vi "UIntToDouble.vi"(1 "Value":u32, 2 "Max":dbl, 3 "Min":dbl) -> (0 "Number":dbl)   [LabVIEW 2009]
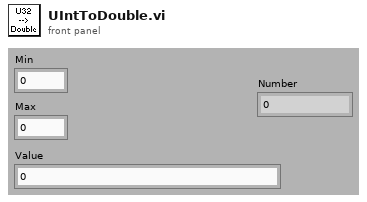
[diagram p1: front panel]
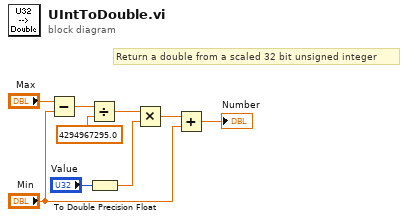
[diagram p0: block diagram]
diagram:
  # "Return a double from a scaled 32 bit unsigned integer"
  n1 = Subtract(x="Max", y="Min") -> (x-y=w9:dbl)
  n2 = Divide(x=w9, y=4294967295.0) -> (x/y=w6:dbl)
  n3 = To Double Precision Float(number="Value") -> (double precision float=w4:dbl)
  n4 = Multiply(x=w6, y=w4) -> (x*y=w3:dbl)
  n5 = Add(x=w3, y="Min") -> (x+y=→"Number":dbl)
